vi "Do.vi"(8 "error in (no error)":errorcluster, 10 "Actor in":refnum<class "Actor.lvclass">, 11 "Stop Event Message":refnum<class "Stop Event Message.lvclass">) -> (0 "error out":errorcluster, 2 "Actor out":refnum<class "Actor.lvclass">)   [LabVIEW 2017, in "Stop Event Message.lvclass"]
doc: "(<B>Filename</B>: Actor Framework.lvlib:Message.lvclass:Do.vi)\n\nDefines what a message does when it is received by an actor. Generally, a message instructs an actor to invoke one of its methods. By default, this method does nothing. A child class must override it to define behavior. Create a child class by using the Actor Framework Message Maker dialog box."
uses:
  Stop Event Message.lvclass
  <vilib>/ActorFramework/Actor/Actor.lvclass
  StopEnabledActor.lvclass
  C:/Program Files (x86)/National Instruments/LabVIEW 2017/vi.lib/ActorFramework/Actor/Actor.lvclass
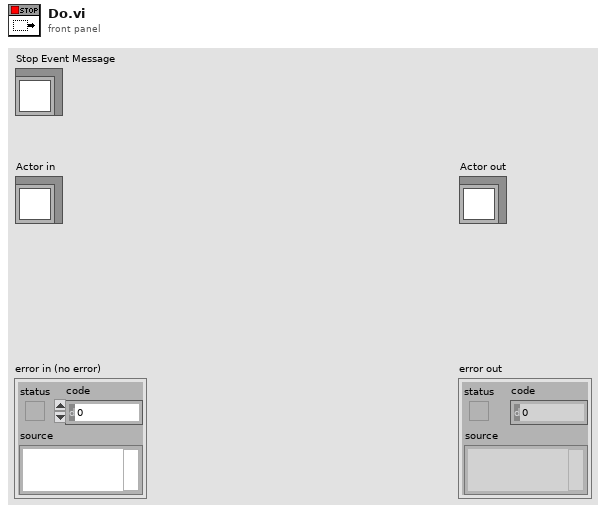
[diagram p1: front panel]
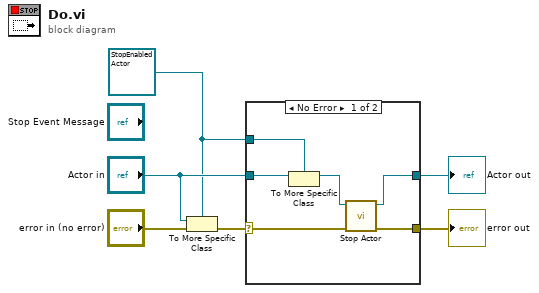
[diagram p0: block diagram]
diagram:
  w4 = refnum<class "StopEnabledActor.lvclass"> refnum ("StopEnabledActor.lvclass")
  n1 = To More Specific Class(target class=w4, reference="Actor in", error in="error in (no error)") -> (error out=w6:errorcluster)  [unwired: 1 out]
  n2 = case shown="No Error" w6 {
    selector: w6 -> [w9 w13]
    tunnel: "Actor in" -> [w12 w14]
    tunnel: w4 -> [w11 _]
    tunnel: [w8 w13] -> w3
    tunnel: [w7 w14] -> w2
    frame No Error {
      n3 = To More Specific Class(target class=w11, reference=w12) -> (specific class reference=w10:refnum<class "StopEnabledActor.lvclass">)  [unwired: 1 in, 1 out]
      n4 = call "Stop Actor.vi"("error in (no error)"=w9, "StopEnabledActor in"=w10) -> ("error out"=w8:errorcluster, "StopEnabledActor out"=w7:refnum<class "StopEnabledActor.lvclass">)  [unwired: 8 in]
    }
    frame Error {
    }
  }
  "error out" <- w3
  "Actor out" <- w2
